vi "_RT_CtrlLoop_Laser_Check_QMark.vi"(1 "ReadValue_String":string) -> (0 "Is Exist?":bool)   [LabVIEW 2018]
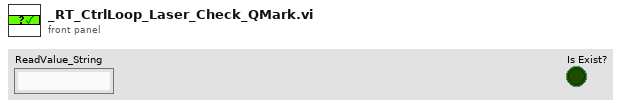
[diagram p1: front panel]
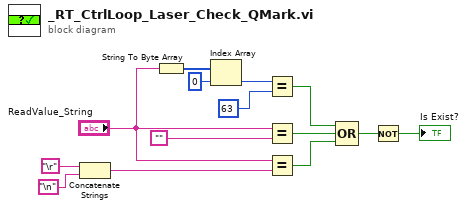
[diagram p0: block diagram]
diagram:
  n1 = Concatenate Strings("\r", "\n") -> (w12:string)
  n2 = String To Byte Array(string="ReadValue_String") -> (unsigned byte array=w11:u8[])
  n3 = Index Array(array=w11, index=0) -> (element=w9:u8)
  n4 = Equal?(x=w9, y=u8 63) -> (x = y?=w4:bool)
  n5 = Equal?(x="ReadValue_String", y="") -> (x = y?=w5:bool)
  n6 = Equal?(x="ReadValue_String", y=w12) -> (x = y?=w3:bool)
  n7 = Compound Arithmetic op=OR(w4, w5, w3) -> (w2:bool)
  n8 = Not(x=w2) -> (.not. x?=→"Is Exist?":bool)
